vi "RxAM.vi"() -> ()   [LabVIEW 2012]
uses:
  <instrlib>/niUSRP/niUSRP Fetch Rx Data (CDB WDT).vi
  <vilib>/Analysis/3filter.llb/Filter Passband Type.ctl
  <vilib>/Analysis/NI_AALBase.lvlib
  <vilib>/measure/NI_MAPro.lvlib
  <vilib>/Analysis/3filter.llb/Butterworth Filter (DBL).vi
  <vilib>/measure/maspectr.llb/FFT Power Spectrum and PSD for 1 Chan.vi
panel:
  out "Power Spectrum":cluster{"f0":dbl, "df":dbl, "magnitude":dbl[]}(graph)
  out "Baseband Output":dbl[](graph)
  in  "stop":bool
  out "error out":errorcluster
  in  "number of samples":i64=200000
  in  "active antenna":string="RX2"
  out "actual gain (dB)":dbl format="%#_6f"
  in  "gain (dB)":dbl format="%#_6f"
  out "actual carrier frequency":dbl=100000.0 format="%#_6p"
  in  "carrier frequency":dbl=915000000.0 format="%#_6p"
  out "actual IQ rate":dbl=100000.0 format="%#_6p"
  in  "IQ rate":dbl=1000000.0 format="%#_6p"
  in  "device names":refnum<k15>="192.168.10.2"
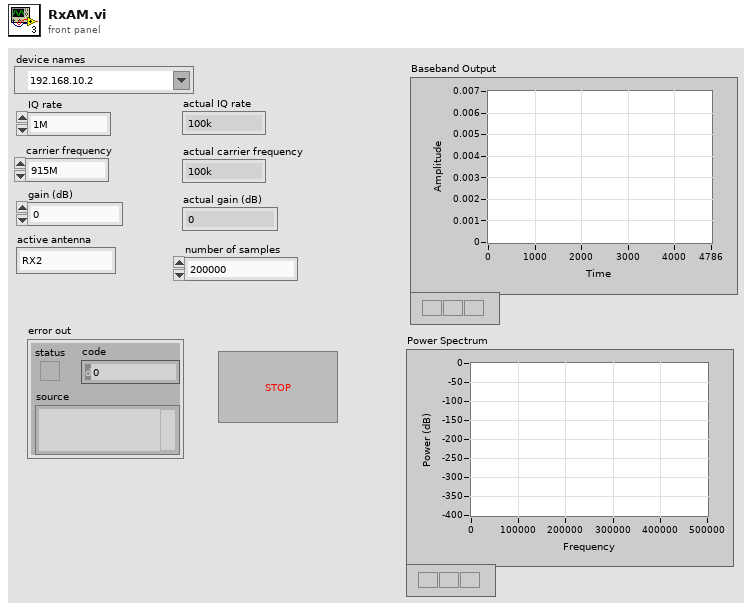
[diagram p1: front panel]
types:
  T1 = typedef "NI_AALBase.lvlib/Filter Passband Type.ctl" = enum32{"Lowpass", "Highpass", "Bandpass", "Bandstop"}
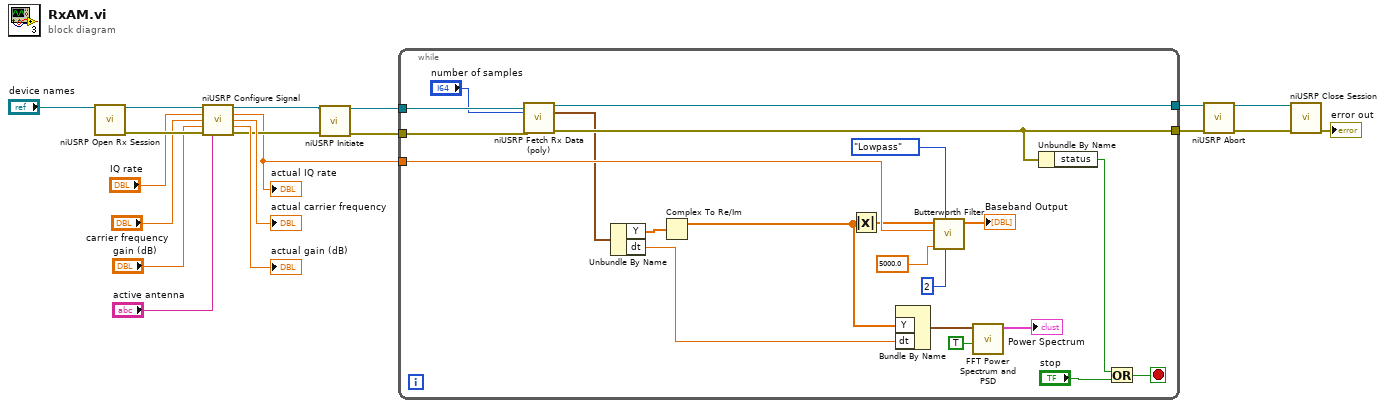
[diagram p0: block diagram]
diagram:
  n1 = call <instrlib>:"niUSRP Open Rx Session.vi"("device names"="device names") -> ("session handle out"=w18:refnum<k15>, "error out"=w17:errorcluster)  [unwired: 13 in]
  n2 = call <instrlib>:"niUSRP Configure Signal.vi"("session handle"=w18, "IQ rate"="IQ rate", "carrier frequency"="carrier frequency", "gain"="gain (dB)", "error in (no error)"=w17, "active antenna"="active antenna") -> ("session handle out"=w11:refnum<k15>, "coerced IQ rate"=w1:dbl, "coerced carrier frequency"=→"actual carrier frequency":dbl, "coerced gain"=→"actual gain (dB)":dbl, "error out"=w10:errorcluster)  [unwired: 5 in]
  "actual IQ rate" <- w1
  n3 = call <instrlib>:"niUSRP Initiate.vi"("session handle"=w11, "error in (no error)"=w10) -> ("session handle out"=w8:refnum<k15>, "error out"=w7:errorcluster)  [unwired: 12 in]
  n4 = while {
    tunnel: w8 -> [w40]
    tunnel: w7 -> [w39]
    tunnel: [w38] -> w6
    tunnel: [w34] -> w5
    tunnel: w1 -> [w27]
    stop <- w37 stop-if-true
    n5 = call-poly <instrlib>:"niUSRP Fetch Rx Data (poly).vi"("session handle"=w40, "number of samples"="number of samples", "error in (no error)"=w39) -> ("session handle out"=w38:refnum<k15>, "data"=w22:waveform(cdb), "error out"=w34:errorcluster)  [unwired: 9 in, 1 out]
    n6 = Unbundle By Name(w22) -> ("Y"=w30:cdb[], "dt"=w23:dbl)
    n7 = Complex To Re/Im(x + iy=w30) -> (x=w20:dbl[])  [unwired: 1 out]
    n8 = Absolute Value(x=w20) -> (abs(x)=w25:dbl[])
    n9 = Bundle By Name("Y"=w20, "dt"=w23) -> (w21:waveform(dbl))  [unwired: 1 in]
    n10 = call-poly <vilib>:"Butterworth Filter.vi"("order"=2, "filter type"=Filter_Passband_Type."Lowpass", "low cutoff freq: fl"=5000.0, "sampling freq: fs"=w27, "X"=w25) -> ("Filtered X"=→"Baseband Output":dbl[])  [unwired: 3 in, 1 out]
    n11 = call-poly <vilib>:"FFT Power Spectrum and PSD.vi"("dB On (F)"=TRUE, "time signal"=w21) -> ("Power Spectrum / PSD"=→"Power Spectrum":cluster{"f0":dbl, "df":dbl, "magnitude":dbl[]})  [unwired: 6 in, 3 out]
    n12 = Unbundle By Name(w34) -> ("status"=w36:bool)
    n13 = Or(x=w36, y="stop") -> (x .or. y?=w37:bool)
  }
  n14 = call <instrlib>:"niUSRP Abort.vi"("session handle"=w6, "error in (no error)"=w5) -> ("session handle out"=w4:refnum<k15>, "error out"=w3:errorcluster)  [unwired: 12 in]
  n15 = call <instrlib>:"niUSRP Close Session.vi"("session handle"=w4, "error in (no error)"=w3) -> ("error out"=→"error out":errorcluster)  [unwired: 13 in]
